vi "field_sweep_2.vi"() -> ()   [LabVIEW 2016]
uses:
  Controls/State.ctl
  Controls/Data.ctl
  <vilib>/Utility/error.llb/DialogType.ctl
  <vilib>/DAQmx/write.llb/DAQmx Write (Analog DBL 1Chan 1Samp).vi
  <vilib>/DAQmx/create/channels.llb/DAQmx Create Channel (AO-Voltage-Basic).vi
  <vilib>/DAQmx/miscellaneous.llb/DAQmx Fill In Error Info.vi
  <instrlib>/niVNA/niVNA.llb/niVNA Fetch Sweep Measurement (DBL).vi
panel:
  in  "Clear button":bool
  in  "Hysteresis":bool caption="Hysteresis On/Off"
  out "DAQ channel Out":tag="DAQ_6363/ao1"
  in  "Averaging Points":i32=10 min=1 max=3201 step=1
  in  "DAQ channel In":tag="DAQ_6363/ao1"
  in  "Exit Button":bool
  in  "IF Bandwidth":dbl(ring)=1000.0 items=["10 Hz"=10.0, "30 Hz"=30.0, "100 Hz"=100.0, "300 Hz"=300.0, "1 KHz"=1000.0, "3 KHz"=3000.0, "10 KHz"=10000.0, "30 KHz"=30000.0]
  in  "Speed (Oe/sec)":dbl=5.0
  in  "Frequency (Hz)":dbl=3000000000.0 min=10000000.0 max=6000000000.0
  in  "Save Button":bool
  out "Status":string="Shutting down...Sweeping field to zero..."
  out "Cursor":cluster{"x":dbl, "y":dbl} {"x" format="%.2f"; "y" format="%.5f"}
  out "VNA Name Out":refnum<k15>="VNA_5630"
  out "Error Out":errorcluster
  in  "Error In (no error)":errorcluster
  in  "Format":i32(ring)=1 items=["Log Magnitude (dB)"=0, "Lin Magnitude"=1, "Phase (deg)"=2, "VSWR"=3, "Group Delay"=6]
  out "SpectrumGraph":cluster{"Old Field":dbl[], "Old Signal":dbl[]}[](graph)
  in  "S-parameter":i32(ring)=1 caption="Measurement" items=["S11", "S21"]
  in  "Start Button":bool
  in  "Stop Button":bool
  in  "Output Power (dBm)":dbl=1.0 min=-25.0 max=5.0 step=0.5
  in  "Number of Points":i32=1000 min=1 max=3201 step=1
  in  "Stop H Field (Oe)":dbl=1500.0 min=-6000.0 max=6000.0 format="%#_6f"
  in  "Start H Field (Oe)":dbl=1000.0 min=-6000.0 max=6000.0 format="%#_6f"
  in  "VNA Name In":refnum<k15>="VNA_5630"
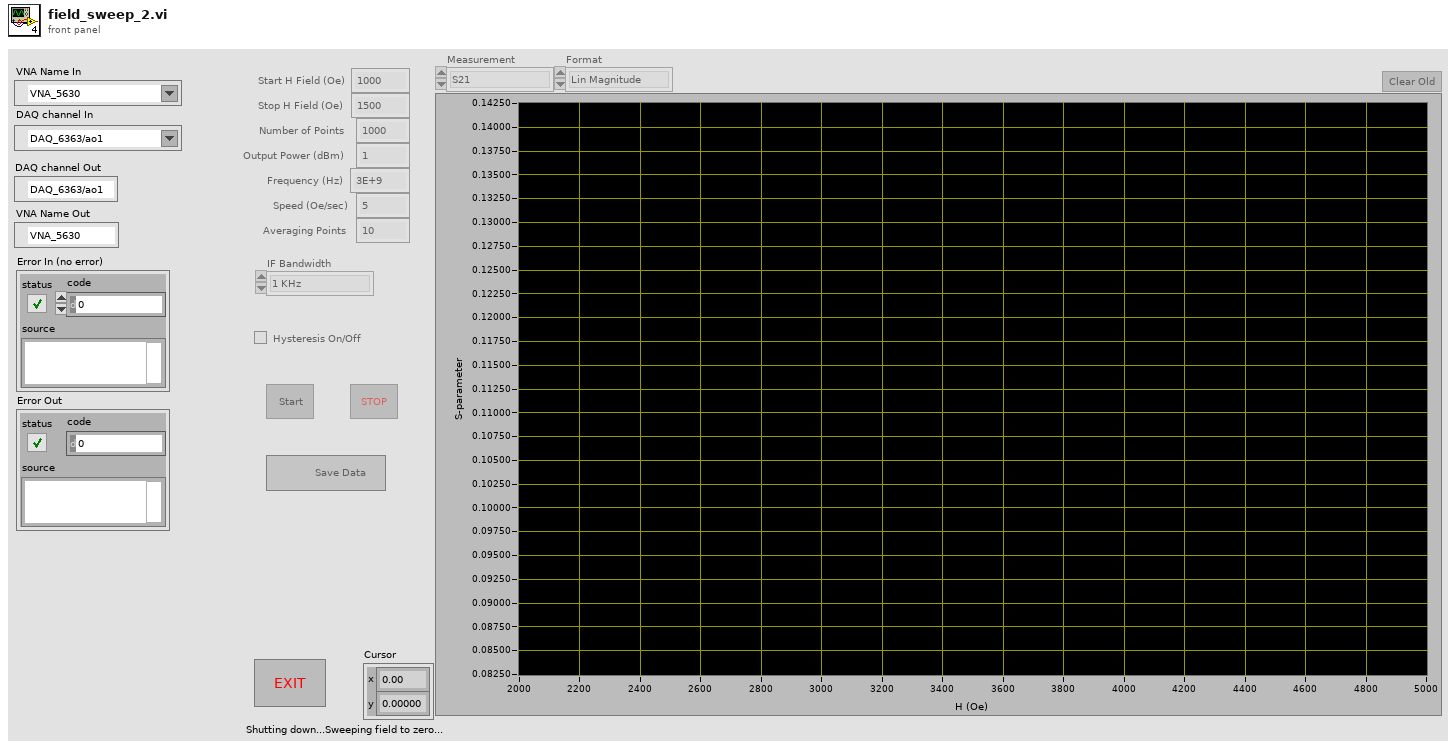
[diagram p1: front panel]
types:
  T1 = typedef "Data.ctl" = cluster{"Field":dbl[], "Signal":dbl[], "Old Field":dbl[], "Old Signal":dbl[]}
  T2 = typedef "State.ctl" = enum16{"Init", "Idle", "Sweeping up", "Sweeping down", "Running", "Running down", "Shutdown"}
  T3 = typedef "DialogType.ctl" = u16
  T4 = typedef "LVPoint32TypeDef.ctl" = cluster{"Horizontal":i32, "Vertical":i32}
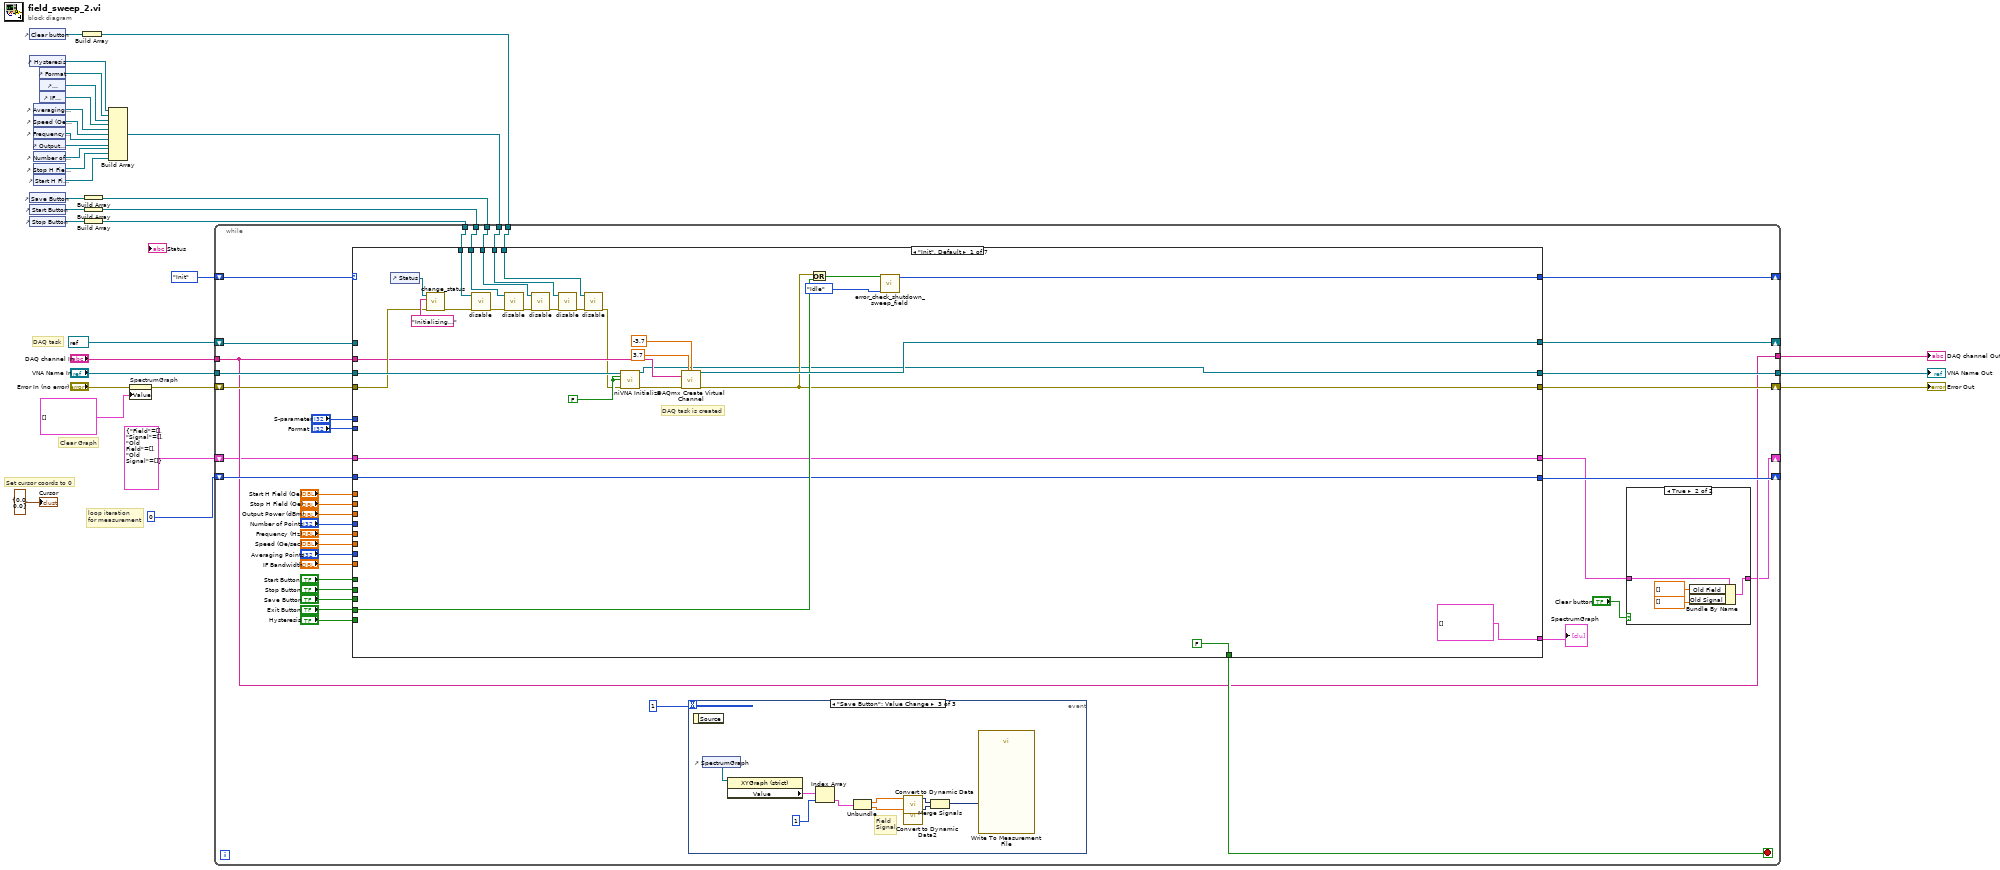
[diagram p0: block diagram]
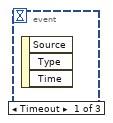
[diagram p3: hidden frame]
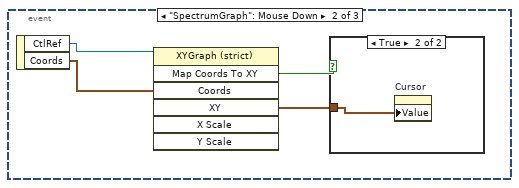
[diagram p4: hidden frame]
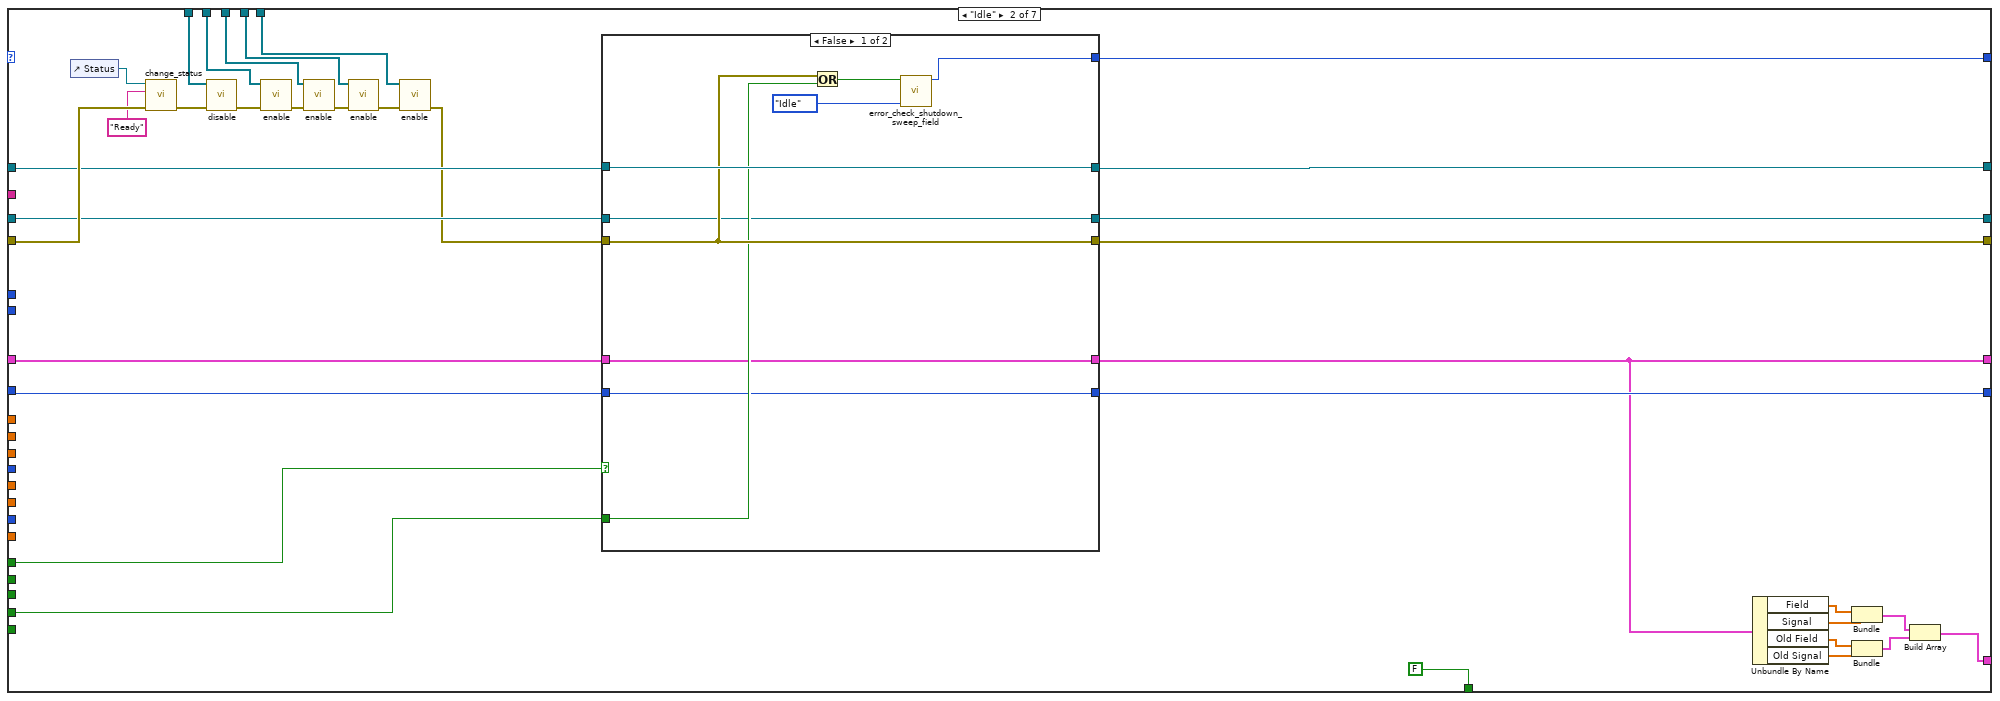
[diagram p6: hidden frame]
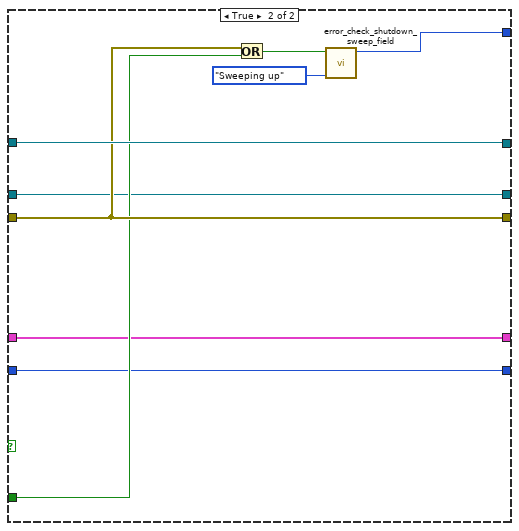
[diagram p7: hidden frame]
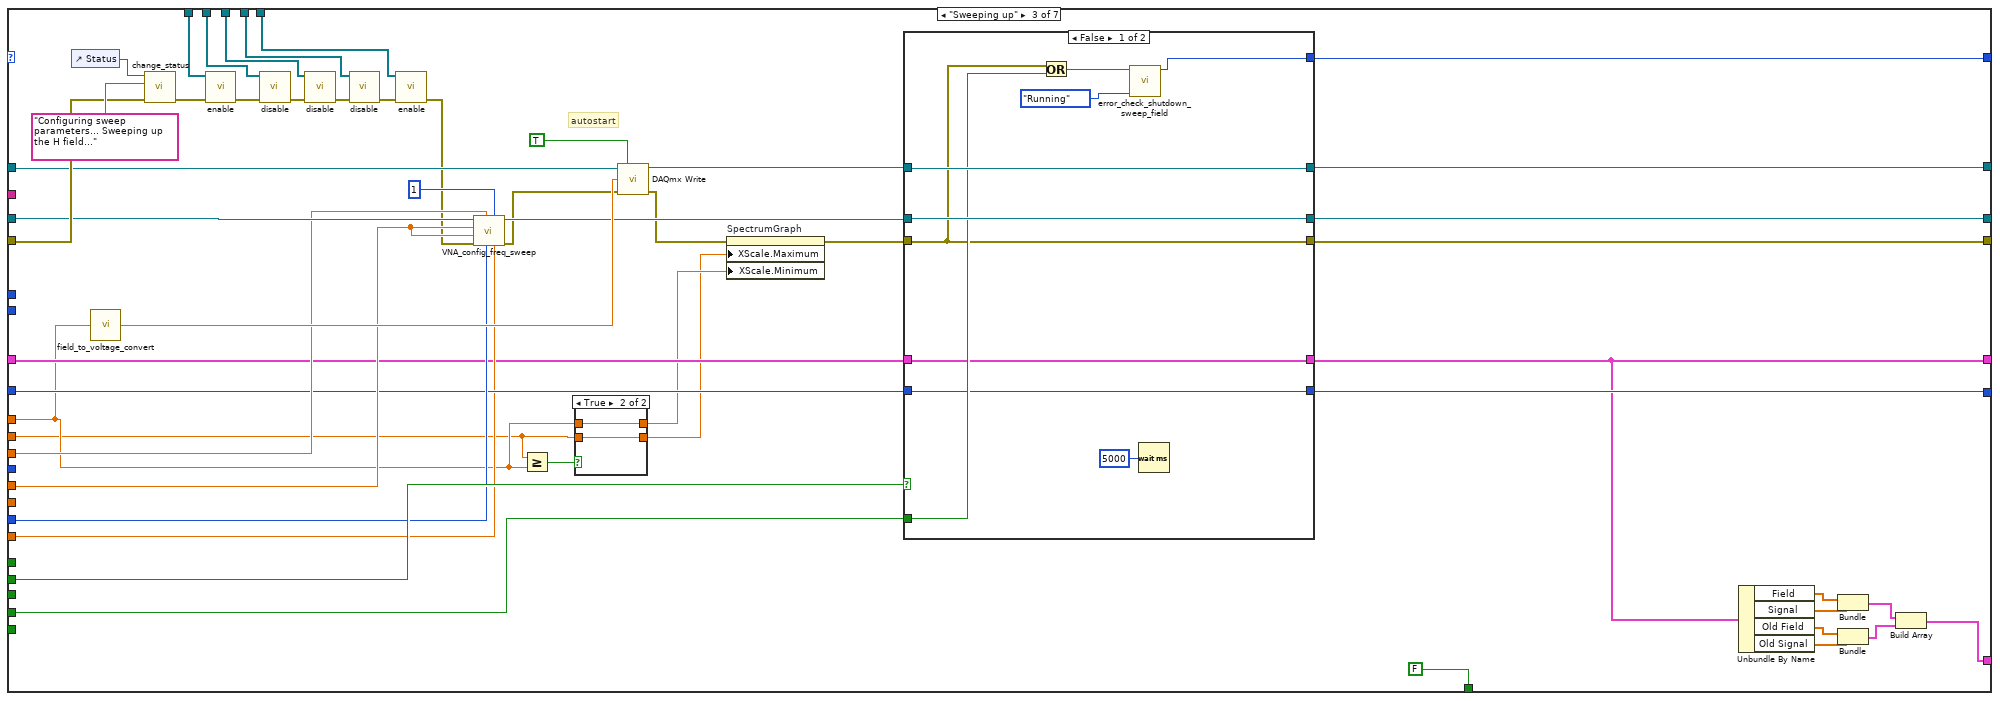
[diagram p8: hidden frame]
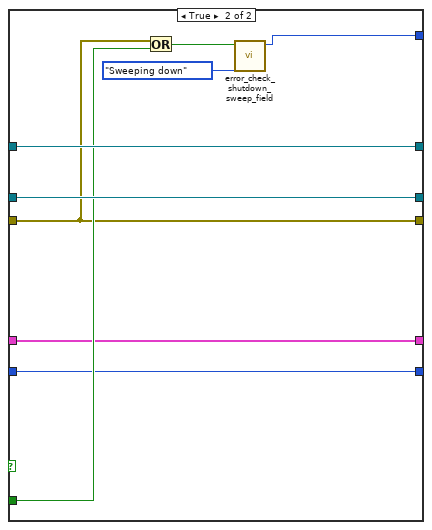
[diagram p10: hidden frame]
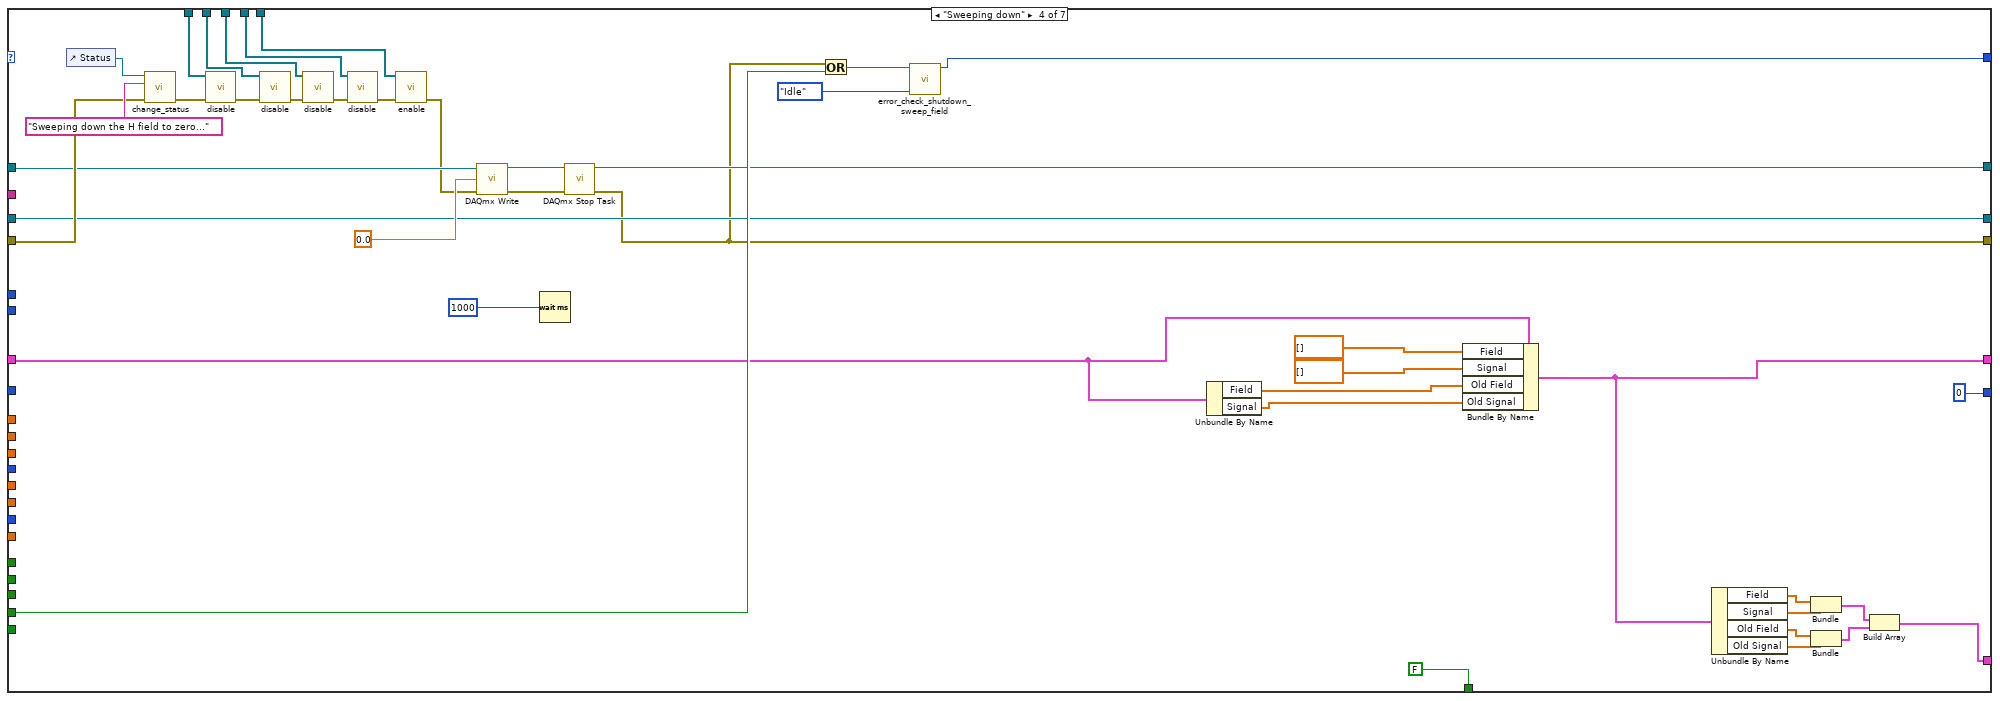
[diagram p11: hidden frame]
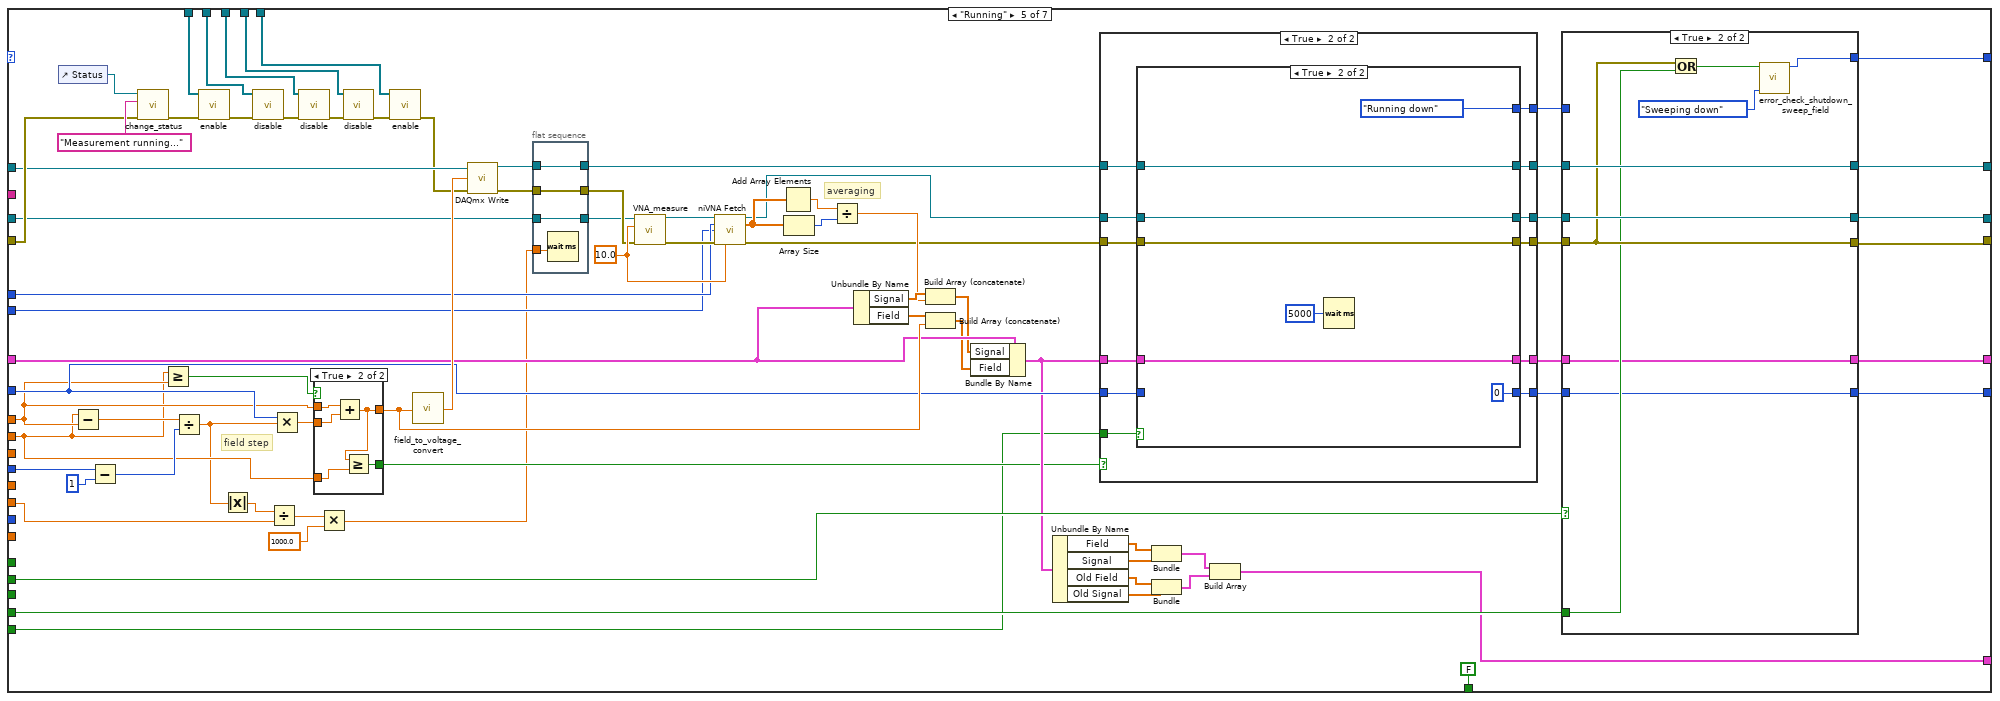
[diagram p12: hidden frame]
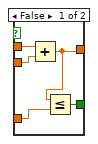
[diagram p13: hidden frame]
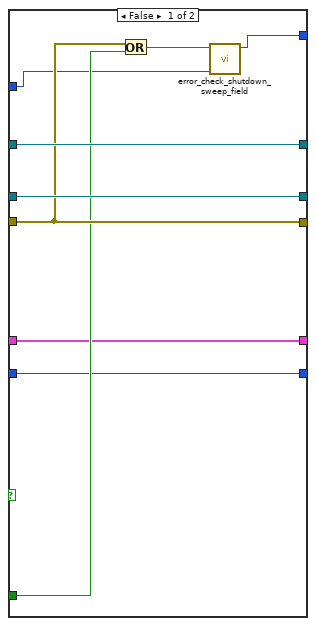
[diagram p14: hidden frame]
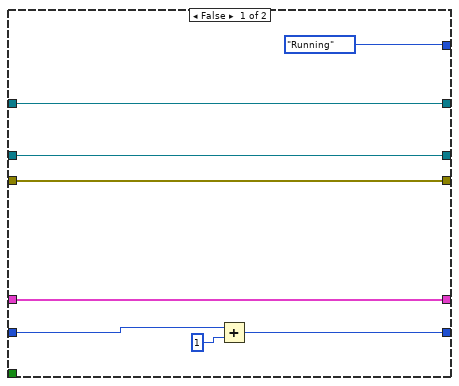
[diagram p15: hidden frame]
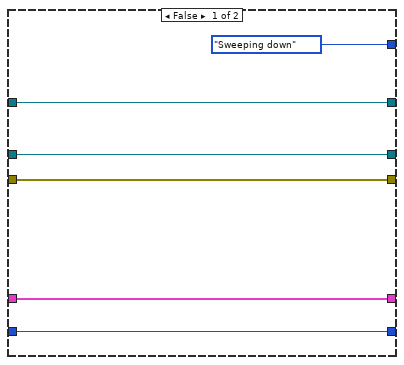
[diagram p16: hidden frame]
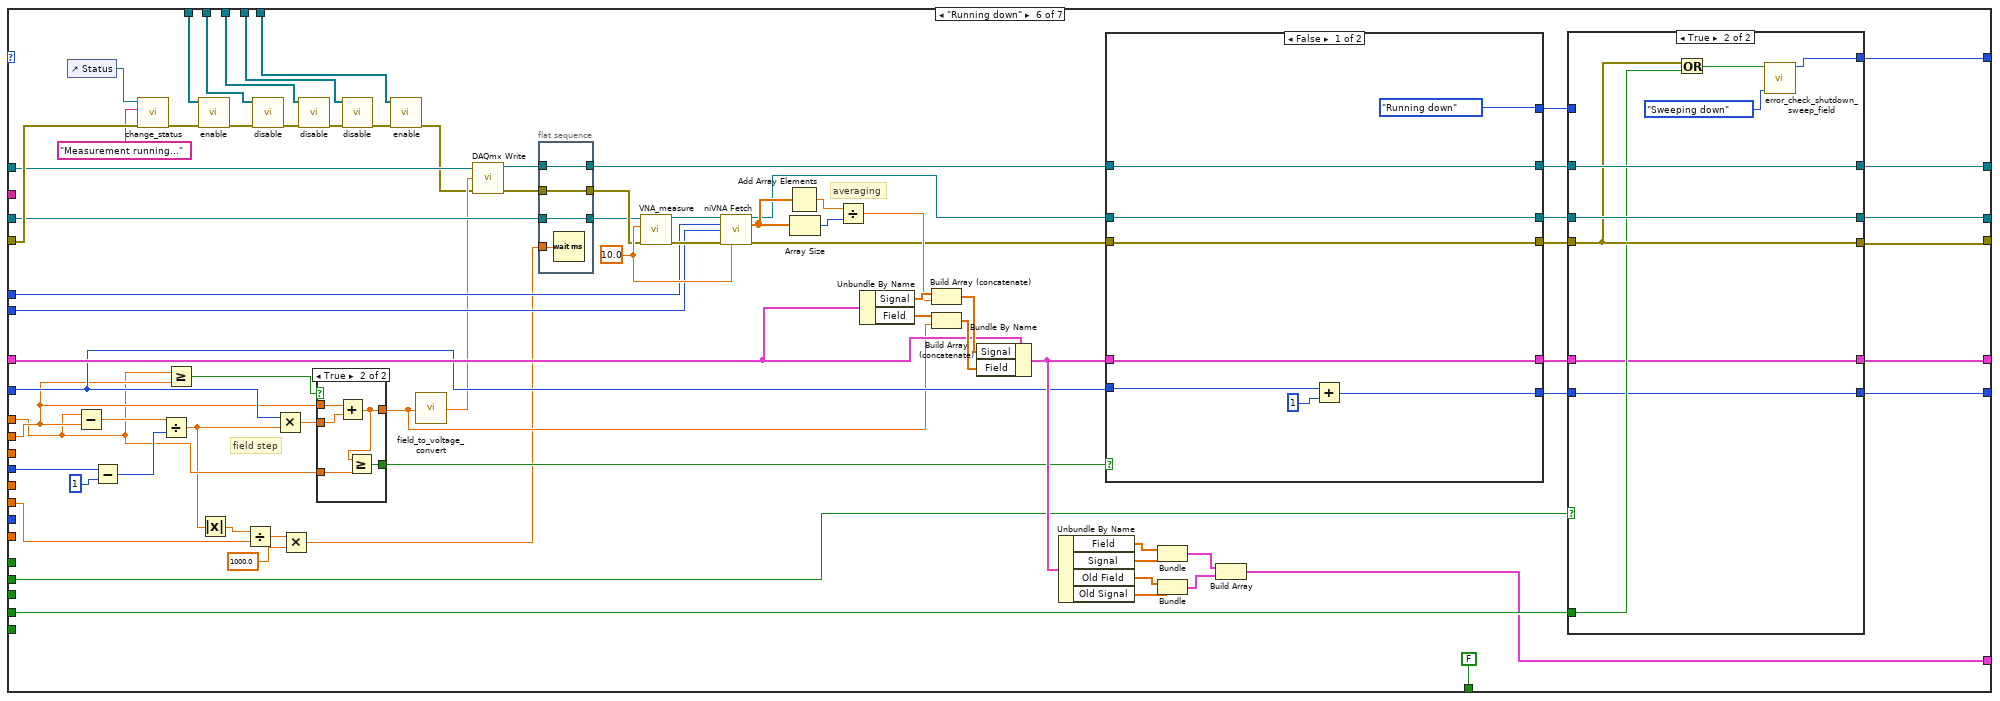
[diagram p17: hidden frame]
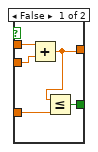
[diagram p18: hidden frame]
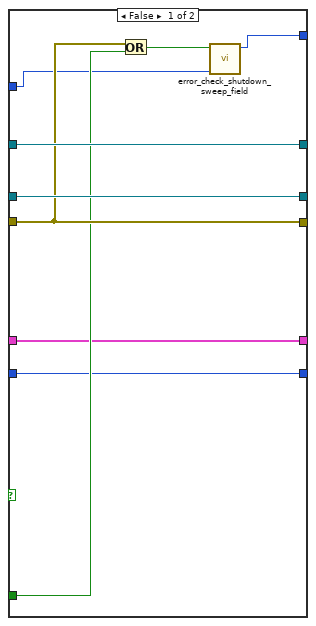
[diagram p19: hidden frame]
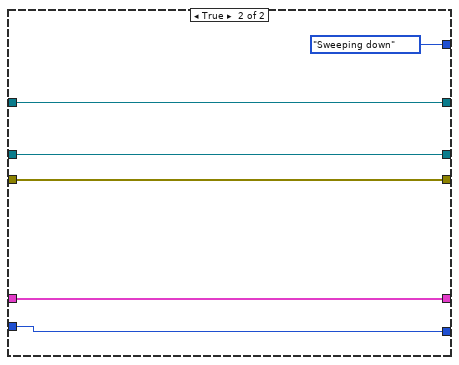
[diagram p20: hidden frame]
diagram:
  # "loop iteration\nfor measurement"
  # "DAQ task"
  # "Set cursor coords to 0"
  # "Clear Graph"
  n1 = control-ref of="Clear button"() -> (w2:refnum<vi>)
  n2 = control-ref of="Hysteresis"() -> (w3:refnum<vi>)
  n3 = control-ref of="Save Button"() -> (w16:refnum<vi>)
  n4 = control-ref of="Start Button"() -> (w24:refnum<vi>)
  n5 = control-ref of="Stop Button"() -> (w23:refnum<vi>)
  n6 = control-ref of="Averaging Points"() -> (w13:refnum<vi>)
  n7 = control-ref of="Speed (Oe/sec)"() -> (w30:refnum<vi>)
  n8 = control-ref of="Frequency (Hz)"() -> (w29:refnum<vi>)
  n9 = control-ref of="Output Power (dBm)"() -> (w28:refnum<vi>)
  n10 = control-ref of="Number of Points"() -> (w27:refnum<vi>)
  n11 = control-ref of="Stop H Field (Oe)"() -> (w26:refnum<vi>)
  n12 = control-ref of="Start H Field (Oe)"() -> (w25:refnum<vi>)
  n13 = control-ref of="Format"() -> (w4:refnum<vi>)
  n14 = control-ref of="S-parameter"() -> (w5:refnum<vi>)
  n15 = control-ref of="IF Bandwidth"() -> (w31:refnum<vi>)
  n16 = Build Array(w2) -> (w1:refnum<vi>[])
  n17 = Build Array(w16) -> (w15:refnum<vi>[])
  n18 = Build Array(w24) -> (w21:refnum<vi>[])
  n19 = Build Array(w23) -> (w20:refnum<vi>[])
  n20 = Build Array(w3, w4, w5, w31, w13, w30, w29, w28, w27, w26, w25) -> (w22:refnum<vi>[])
  n21 = property on="SpectrumGraph" class="XYGraph (strict)"(error in="Error In (no error)", "Value"=cluster{"Old Field":dbl[], "Old Signal":dbl[]}[] [] ("SpectrumGraph")) -> (error out=w9:errorcluster)  [unwired: 1 in, 1 out]
  n22 = while {
    shift-right: [w66] -> _
    shift-left: State."Init" -> [w71]
    shift-right: [w46] -> _
    shift-left: 0 -> [w48]
    tunnel: w22 -> [w70]
    tunnel: w21 -> [w69]
    tunnel: w20 -> [w68]
    tunnel: "VNA Name In" -> [w67]
    tunnel: "DAQ channel In" -> [w45]
    shift-right: [w65] -> w6
    shift-left: w9 -> [w64]
    shift-right: [w63] -> _
    shift-left: refnum<k21> refnum ("task in") -> [w62]
    tunnel: w15 -> [w61]
    tunnel: [w49] -> w12
    shift-right: [w35] -> _
    shift-left: T1 {"Field"=[], "Signal"=[], "Old Field"=[], "Old Signal"=[]} ("Cluster") -> [w42]
    tunnel: [w45] -> w11
    tunnel: w1 -> [w34]
    stop <- w56 stop-if-true
    n23 = case shown="\"Init\", Default" w71 {
      tunnel: w70 -> [w106 w152 w216 w280 w359 w500 w585]
      tunnel: w69 -> [w119 w154 w218 w278 w361 w502 w587]
      tunnel: w68 -> [w121 w155 w219 w277 w363 w503 w588]
      tunnel: w67 -> [w114 w142 w205 w273 w334 w472 w570]
      tunnel: w64 -> [w113 w147 w214 w283 w357 w506 w583]
      tunnel: [w102 w139 w207 w274 w318 w456 State."Shutdown"] -> w66
      tunnel: w45 -> [w109 _ _ _ _ _ _]
      tunnel: [w101 w143 w212 w266 w324 w458 w578] -> w65
      tunnel: [w108 w140 w210 w268 w328 w457 w579] -> w63
      tunnel: w62 -> [_ w141 w192 w281 w356 w473 w573]
      tunnel: w61 -> [w107 w153 w217 w279 w360 w501 w586]
      tunnel: "Start Button" -> [_ w144 _ _ _ _ _]
      tunnel: "Stop Button" -> [_ _ w213 _ w323 w469 _]
      tunnel: "Save Button" -> [_ _ _ _ _ _ _]
      tunnel: "Exit Button" -> [w103 w138 w206 w275 w322 w462 _]
      tunnel: [FALSE FALSE FALSE FALSE FALSE FALSE TRUE] -> w56
      tunnel: "Start H Field (Oe)" -> [_ _ w188 _ w304 w445 _]
      tunnel: "Stop H Field (Oe)" -> [_ _ w187 _ w302 w446 _]
      tunnel: "Output Power (dBm)" -> [_ _ w202 _ _ _ _]
      tunnel: "Number of Points" -> [_ _ _ _ w345 w449 _]
      tunnel: "Frequency (Hz)" -> [_ _ w203 _ _ _ _]
      tunnel: "Speed (Oe/sec)" -> [_ _ _ _ w346 w438 _]
      tunnel: [w99 w137 w211 w273 w326 w459 w580] -> w49
      tunnel: w48 -> [w98 w135 w200 _ w330 w450 w568]
      tunnel: "Averaging Points" -> [_ _ w201 _ _ _ _]
      tunnel: [w98 w136 w199 0 w320 w460 w568] -> w46
      tunnel: "IF Bandwidth" -> [_ _ w195 _ _ _ _]
      tunnel: [w96 w125 w177 w251 w312 w461 T1 {"Field"=[], "Signal"=[], "Old Field"=[], "Old Signal"=[]} ("Cluster")] -> w36
      tunnel: w42 -> [w96 w133 w193 w262 w316 w468 _]
      tunnel: "Hysteresis" -> [_ _ _ _ w300 _ _]
      tunnel: "S-parameter" -> [_ _ _ _ w299 w471 _]
      tunnel: "Format" -> [_ _ _ _ w298 w470 _]
      tunnel: [cluster{"Old Field":dbl[], "Old Signal":dbl[]}[] [] w126 w178 w252 w297 w444 cluster{"Old Field":dbl[], "Old Signal":dbl[]}[] []] -> w38
      tunnel: w34 -> [w92 w123 w175 w249 w289 w434 w558]
      frame "Init", Default {
        w115 = FALSE ("id query")
        # "DAQ task is created"
        n24 = control-ref of="Status"() -> (w117:refnum<vi>)
        n25 = call "change_status.vi"("error in (no error)"=w113, "String"="Initializing...", "String in"=w117) -> ("error out"=w118:errorcluster)  [unwired: 8 in]
        n26 = call "disable.vi"("error in (no error)"=w118, "Array"=w121) -> ("error out"=w120:errorcluster)  [unwired: 9 in]
        n27 = call "disable.vi"("error in (no error)"=w120, "Array"=w119) -> ("error out"=w105:errorcluster)  [unwired: 9 in]
        n28 = call "disable.vi"("error in (no error)"=w105, "Array"=w107) -> ("error out"=w104:errorcluster)  [unwired: 9 in]
        n29 = call "disable.vi"("error in (no error)"=w104, "Array"=w106) -> ("error out"=w93:errorcluster)  [unwired: 9 in]
        n30 = call "disable.vi"("error in (no error)"=w93, "Array"=w92) -> ("error out"=w91:errorcluster)  [unwired: 9 in]
        n31 = call <instrlib>:"niVNA Initialize.vi"("resource name"=w114, "id query"=w115, "reset"=w115, "error in"=w91) -> ("instrument handle"=w99:refnum<k15>, "error out"=w112:errorcluster)  [unwired: 10 in]
        n32 = call-poly <vilib>:"DAQmx Create Virtual Channel.vi"("maximum value"=3.7, "minimum value"=-3.7, "physical channels"=w109, "error in"=w112) -> ("task out"=w108:refnum<k21>, "error out"=w101:errorcluster)  [unwired: 10 in]
        n33 = Or(x=w101, y=w103) -> (x .or. y?=w100:bool)
        n34 = call "error_check_shutdown_sweep_field.vi"("State In"=State."Idle", "Boolean"=w100) -> ("State Out"=w102:T2)  [unwired: 9 in]
      }
      frame "Idle" {
        n35 = control-ref of="Status"() -> (w146:refnum<vi>)
        n36 = call "change_status.vi"("error in (no error)"=w147, "String"="Ready", "String in"=w146) -> ("error out"=w148:errorcluster)  [unwired: 8 in]
        n37 = call "disable.vi"("error in (no error)"=w148, "Array"=w155) -> ("error out"=w151:errorcluster)  [unwired: 9 in]
        n38 = call "enable.vi"("error in (no error)"=w151, "Array"=w154) -> ("error out"=w150:errorcluster)  [unwired: 9 in]
        n39 = call "enable.vi"("error in (no error)"=w150, "Array"=w153) -> ("error out"=w149:errorcluster)  [unwired: 9 in]
        n40 = call "enable.vi"("error in (no error)"=w149, "Array"=w152) -> ("error out"=w124:errorcluster)  [unwired: 9 in]
        n41 = call "enable.vi"("error in (no error)"=w124, "Array"=w123) -> ("error out"=w122:errorcluster)  [unwired: 9 in]
        n42 = case shown="False" w144 {
          tunnel: w122 -> [w161 w171]
          tunnel: [w161 w171] -> w143
          tunnel: w142 -> [w159 w168]
          tunnel: w141 -> [w164 w173]
          tunnel: [w164 w173] -> w140
          tunnel: [w162 w169] -> w139
          tunnel: w138 -> [w160 w170]
          tunnel: [w159 w168] -> w137
          tunnel: [w158 w167] -> w136
          tunnel: w135 -> [w158 w167]
          tunnel: w133 -> [w157 w166]
          tunnel: [w157 w166] -> w125
          frame False {
            n43 = Or(x=w161, y=w160) -> (x .or. y?=w163:bool)
            n44 = call "error_check_shutdown_sweep_field.vi"("State In"=State."Idle", "Boolean"=w163) -> ("State Out"=w162:T2)  [unwired: 9 in]
          }
          frame True {
            n45 = Or(x=w171, y=w170) -> (x .or. y?=w172:bool)
            n46 = call "error_check_shutdown_sweep_field.vi"("State In"=State."Sweeping up", "Boolean"=w172) -> ("State Out"=w169:T2)  [unwired: 9 in]
          }
        }
        n47 = Unbundle By Name(w125) -> ("Field"=w132:dbl[], "Signal"=w131:dbl[], "Old Field"=w130:dbl[], "Old Signal"=w129:dbl[])
        n48 = Bundle("Field"=w132, "Signal"=w131) -> (w128:cluster{"Field":dbl[], "Signal":dbl[]})  [unwired: 1 in]
        n49 = Bundle("Old Field"=w130, "Old Signal"=w129) -> (w127:cluster{"Old Field":dbl[], "Old Signal":dbl[]})  [unwired: 1 in]
        n50 = Build Array(w128, w127) -> (w126:cluster{"Old Field":dbl[], "Old Signal":dbl[]}[])
      }
      frame "Sweeping up" {
        # "autostart"
        n51 = control-ref of="Status"() -> (w215:refnum<vi>)
        n52 = call "field_to_voltage_convert.vi"("Start H Field (Oe)"=w188) -> ("Numeric"=w208:dbl)
        n53 = call "change_status.vi"("error in (no error)"=w214, "String"="Configuring sweep parameters... Sweeping up the H field...", "String in"=w215) -> ("error out"=w223:errorcluster)  [unwired: 8 in]
        n54 = call "enable.vi"("error in (no error)"=w223, "Array"=w219) -> ("error out"=w222:errorcluster)  [unwired: 9 in]
        n55 = call "disable.vi"("error in (no error)"=w222, "Array"=w218) -> ("error out"=w221:errorcluster)  [unwired: 9 in]
        n56 = call "disable.vi"("error in (no error)"=w221, "Array"=w217) -> ("error out"=w220:errorcluster)  [unwired: 9 in]
        n57 = call "disable.vi"("error in (no error)"=w220, "Array"=w216) -> ("error out"=w176:errorcluster)  [unwired: 9 in]
        n58 = call "enable.vi"("error in (no error)"=w176, "Array"=w175) -> ("error out"=w174:errorcluster)  [unwired: 9 in]
        n59 = call "VNA_config_freq_sweep.vi"("IF Bandwidth"=w195, "Averaging"=1, "Number of Points"=w201, "Output Power"=w202, "error in (no error)"=w174, "Stop Frequency"=w203, "Start Frequency"=w203, "Resource Name In"=w205) -> ("error out"=w191:errorcluster, "Resource Name Out"=w204:refnum<k15>)  [unwired: 2 in]
        n60 = Greater Or Equal?(x=w187, y=w188) -> (x >= y?=w189:bool)
        n61 = case shown="True" w189 {
          tunnel: w188 -> [w226 w228]
          tunnel: w187 -> [w225 w227]
          tunnel: [w225 w228] -> w186
          tunnel: [w226 w227] -> w185
          frame False {
          }
          frame True {
          }
        }
        n62 = call-poly <vilib>:"DAQmx Write.vi"("task/channels in"=w192, "auto start"=TRUE, "data"=w208, "error in"=w191) -> ("task out"=w209:refnum<k21>, "error out"=w197:errorcluster)  [unwired: 9 in, 1 out]
        n63 = property on="SpectrumGraph" class="XYGraph (strict)"(error in=w197, "XScale.Maximum"=w185, "XScale.Minimum"=w186) -> (error out=w196:errorcluster)  [unwired: 1 in, 1 out]
        n64 = case shown="False" w213 {
          tunnel: w196 -> [w233 w242]
          tunnel: w209 -> [w238 w246]
          tunnel: w204 -> [w237 w247]
          tunnel: [w233 w242] -> w212
          tunnel: [w237 w247] -> w211
          tunnel: [w238 w246] -> w210
          tunnel: [w235 w244] -> w207
          tunnel: w206 -> [w234 w243]
          tunnel: w200 -> [w231 w241]
          tunnel: [w231 w241] -> w199
          tunnel: w193 -> [w230 w240]
          tunnel: [w230 w240] -> w177
          frame False {
            n65 = Or(x=w233, y=w234) -> (x .or. y?=w236:bool)
            n66 = call "error_check_shutdown_sweep_field.vi"("State In"=State."Running", "Boolean"=w236) -> ("State Out"=w235:T2)  [unwired: 9 in]
            n67 = Wait (ms)(milliseconds to wait=u32 5000) -> ()  [unwired: 1 out]
          }
          frame True {
            n68 = Or(x=w242, y=w243) -> (x .or. y?=w245:bool)
            n69 = call "error_check_shutdown_sweep_field.vi"("State In"=State."Sweeping down", "Boolean"=w245) -> ("State Out"=w244:T2)  [unwired: 9 in]
          }
        }
        n70 = Unbundle By Name(w177) -> ("Field"=w184:dbl[], "Signal"=w183:dbl[], "Old Field"=w182:dbl[], "Old Signal"=w181:dbl[])
        n71 = Bundle("Field"=w184, "Signal"=w183) -> (w180:cluster{"Field":dbl[], "Signal":dbl[]})  [unwired: 1 in]
        n72 = Bundle("Old Field"=w182, "Old Signal"=w181) -> (w179:cluster{"Old Field":dbl[], "Old Signal":dbl[]})  [unwired: 1 in]
        n73 = Build Array(w180, w179) -> (w178:cluster{"Old Field":dbl[], "Old Signal":dbl[]}[])
      }
      frame "Sweeping down" {
        n74 = control-ref of="Status"() -> (w272:refnum<vi>)
        n75 = call "change_status.vi"("error in (no error)"=w283, "String"="Sweeping down the H field to zero...", "String in"=w272) -> ("error out"=w287:errorcluster)  [unwired: 8 in]
        n76 = call "disable.vi"("error in (no error)"=w287, "Array"=w277) -> ("error out"=w286:errorcluster)  [unwired: 9 in]
        n77 = call "disable.vi"("error in (no error)"=w286, "Array"=w278) -> ("error out"=w285:errorcluster)  [unwired: 9 in]
        n78 = call "disable.vi"("error in (no error)"=w285, "Array"=w279) -> ("error out"=w284:errorcluster)  [unwired: 9 in]
        n79 = call "disable.vi"("error in (no error)"=w284, "Array"=w280) -> ("error out"=w250:errorcluster)  [unwired: 9 in]
        n80 = call "enable.vi"("error in (no error)"=w250, "Array"=w249) -> ("error out"=w248:errorcluster)  [unwired: 9 in]
        n81 = call-poly <vilib>:"DAQmx Write.vi"("task/channels in"=w281, "data"=0.0, "error in"=w248) -> ("task out"=w269:refnum<k21>, "error out"=w267:errorcluster)  [unwired: 10 in, 1 out]
        n82 = Wait (ms)(milliseconds to wait=u32 1000) -> ()  [unwired: 1 out]
        n83 = call <vilib>:"DAQmx Stop Task.vi"("task/channels in"=w269, "error in"=w267) -> ("task out"=w268:refnum<k21>, "error out"=w266:errorcluster)  [unwired: 12 in]
        n84 = Or(x=w266, y=w275) -> (x .or. y?=w276:bool)
        n85 = call "error_check_shutdown_sweep_field.vi"("State In"=State."Idle", "Boolean"=w276) -> ("State Out"=w274:T2)  [unwired: 9 in]
        n86 = Unbundle By Name(w262) -> ("Field"=w261:dbl[], "Signal"=w260:dbl[])
        n87 = Bundle By Name(cluster=w262, "Field"=dbl[] [], "Signal"=dbl[] [], "Old Field"=w261, "Old Signal"=w260) -> (w251:T1)
        n88 = Unbundle By Name(w251) -> ("Field"=w258:dbl[], "Signal"=w257:dbl[], "Old Field"=w256:dbl[], "Old Signal"=w255:dbl[])
        n89 = Bundle("Field"=w258, "Signal"=w257) -> (w254:cluster{"Field":dbl[], "Signal":dbl[]})  [unwired: 1 in]
        n90 = Bundle("Old Field"=w256, "Old Signal"=w255) -> (w253:cluster{"Old Field":dbl[], "Old Signal":dbl[]})  [unwired: 1 in]
        n91 = Build Array(w254, w253) -> (w252:cluster{"Old Field":dbl[], "Old Signal":dbl[]}[])
      }
      frame "Running" {
        w352 = 10.0 ("timeout")
        # "averaging"
        # "field step"
        n92 = control-ref of="Status"() -> (w358:refnum<vi>)
        n93 = Subtract(x=w302, y=w304) -> (x-y=w340:dbl)
        n94 = Subtract(x=w345, y=1) -> (x-y=w354:i32)
        n95 = call "change_status.vi"("error in (no error)"=w357, "String"="Measurement running...", "String in"=w358) -> ("error out"=w364:errorcluster)  [unwired: 8 in]
        n96 = Greater Or Equal?(x=w302, y=w304) -> (x >= y?=w303:bool)
        n97 = Divide(x=w340, y=w354) -> (x/y=w293:dbl)
        n98 = call "enable.vi"("error in (no error)"=w364, "Array"=w363) -> ("error out"=w367:errorcluster)  [unwired: 9 in]
        n99 = Absolute Value(x=w293) -> (abs(x)=w292:dbl)
        n100 = call "disable.vi"("error in (no error)"=w367, "Array"=w361) -> ("error out"=w366:errorcluster)  [unwired: 9 in]
        n101 = Divide(x=w292, y=w346) -> (x/y=w296:dbl)
        n102 = Multiply(x=w330, y=w293) -> (x*y=w353:dbl)
        n103 = call "disable.vi"("error in (no error)"=w366, "Array"=w360) -> ("error out"=w365:errorcluster)  [unwired: 9 in]
        n104 = case shown="True" w303 {
          tunnel: w353 -> [w371 w377]
          tunnel: w304 -> [w372 w376]
          tunnel: [w369 w374] -> w336
          tunnel: w302 -> [w370 w373]
          tunnel: [w368 w375] -> w301
          frame False {
            n105 = Add(x=w372, y=w371) -> (x+y=w369:dbl)
            n106 = Less Or Equal?(x=w369, y=w370) -> (x <= y?=w368:bool)
          }
          frame True {
            n107 = Add(x=w376, y=w377) -> (x+y=w374:dbl)
            n108 = Greater Or Equal?(x=w374, y=w373) -> (x >= y?=w375:bool)
          }
        }
        n109 = Multiply(x=w296, y=1000.0) -> (x*y=w294:dbl)
        n110 = call "disable.vi"("error in (no error)"=w365, "Array"=w359) -> ("error out"=w291:errorcluster)  [unwired: 9 in]
        n111 = call "enable.vi"("error in (no error)"=w291, "Array"=w289) -> ("error out"=w290:errorcluster)  [unwired: 9 in]
        n112 = call "field_to_voltage_convert.vi"("Start H Field (Oe)"=w336) -> ("Numeric"=w341:dbl)
        n113 = call-poly <vilib>:"DAQmx Write.vi"("task/channels in"=w356, "data"=w341, "error in"=w290) -> ("task out"=w344:refnum<k21>, "error out"=w343:errorcluster)  [unwired: 10 in, 1 out]
        n114 = flat-sequence {
          tunnel: w344 -> [w432]
          tunnel: [w432] -> w335
          tunnel: w343 -> [w431]
          tunnel: [w431] -> w342
          tunnel: w334 -> [w430]
          tunnel: [w430] -> w333
          tunnel: w294 -> [w429]
          frame #0 {
            n115 = Wait (ms)(milliseconds to wait=w429) -> ()  [unwired: 1 out]
          }
        }
        n116 = call "VNA_measure.vi"("error in (no error)"=w342, "timeout"=w352, "Resource Name In"=w333) -> ("error out"=w351:errorcluster, "Resource Name Out"=w350:refnum<k15>)  [unwired: 7 in]
        n117 = call-poly <instrlib>:"niVNA Fetch.vi"("instrument handle"=w350, "measurement"=w299, "format"=w298, "error in"=w351, "timeout"=w352) -> ("instrument handle out"=w332:refnum<k15>, "data"=w349:dbl[], "error out"=w331:errorcluster)  [unwired: 7 in, 1 out]
        n118 = Add Array Elements(numeric array=w349) -> (sum=w348:dbl)
        n119 = Array Size(array=w349) -> (size(s)=w347:i32)
        n120 = Divide(x=w348, y=w347) -> (x/y=w338:dbl)
        n121 = Unbundle By Name(w316) -> ("Signal"=w339:dbl[], "Field"=w337:dbl[])
        n122 = Build Array (concatenate)(w339, w338) -> (w315:dbl[])
        n123 = Build Array (concatenate)(w337, w336) -> (w314:dbl[])
        n124 = Bundle By Name(cluster=w316, "Signal"=w315, "Field"=w314) -> (w311:T1)
        n125 = Unbundle By Name(w311) -> ("Field"=w310:dbl[], "Signal"=w309:dbl[], "Old Field"=w308:dbl[], "Old Signal"=w307:dbl[])
        n126 = case shown="True" w301 {
          tunnel: [State."Running" w415] -> w319
          tunnel: w335 -> [w402 w405]
          tunnel: [w402 w404] -> w329
          tunnel: w332 -> [w401 w407]
          tunnel: [w401 w406] -> w327
          tunnel: w331 -> [w400 w409]
          tunnel: [w400 w408] -> w325
          tunnel: w330 -> [w399 w414]
          tunnel: [w397 w412] -> w321
          tunnel: w311 -> [w396 w411]
          tunnel: [w396 w410] -> w313
          tunnel: w300 -> [_ w413]
          frame False {
            n127 = Add(x=w399, y=1) -> (x+y=w397:i32)
          }
          frame True {
            n128 = case shown="True" w413 {
              tunnel: [State."Sweeping down" State."Running down"] -> w415
              tunnel: w414 -> [w420 _]
              tunnel: [w420 0] -> w412
              tunnel: w411 -> [w419 w425]
              tunnel: [w419 w425] -> w410
              tunnel: w409 -> [w418 w423]
              tunnel: [w418 w423] -> w408
              tunnel: w407 -> [w417 w426]
              tunnel: [w417 w426] -> w406
              tunnel: w405 -> [w416 w427]
              tunnel: [w416 w427] -> w404
              frame False {
              }
              frame True {
                n129 = Wait (ms)(milliseconds to wait=u32 5000) -> ()  [unwired: 1 out]
              }
            }
          }
        }
        n130 = Bundle("Field"=w310, "Signal"=w309) -> (w306:cluster{"Field":dbl[], "Signal":dbl[]})  [unwired: 1 in]
        n131 = Bundle("Old Field"=w308, "Old Signal"=w307) -> (w305:cluster{"Old Field":dbl[], "Old Signal":dbl[]})  [unwired: 1 in]
        n132 = Build Array(w306, w305) -> (w297:cluster{"Old Field":dbl[], "Old Signal":dbl[]}[])
        n133 = case shown="True" w323 {
          tunnel: [w385 w394] -> w318
          tunnel: w329 -> [w384 w393]
          tunnel: [w384 w393] -> w328
          tunnel: w327 -> [w383 w392]
          tunnel: [w383 w392] -> w326
          tunnel: w325 -> [w382 w391]
          tunnel: [w382 w391] -> w324
          tunnel: w322 -> [w381 w390]
          tunnel: w321 -> [w380 w389]
          tunnel: [w380 w389] -> w320
          tunnel: w319 -> [w378 _]
          tunnel: [w379 w388] -> w312
          tunnel: w313 -> [w379 w388]
          frame False {
            n134 = Or(x=w382, y=w381) -> (x .or. y?=w386:bool)
            n135 = call "error_check_shutdown_sweep_field.vi"("State In"=w378, "Boolean"=w386) -> ("State Out"=w385:T2)  [unwired: 9 in]
          }
          frame True {
            n136 = Or(x=w391, y=w390) -> (x .or. y?=w395:bool)
            n137 = call "error_check_shutdown_sweep_field.vi"("State In"=State."Sweeping down", "Boolean"=w395) -> ("State Out"=w394:T2)  [unwired: 9 in]
          }
        }
      }
      frame "Running down" {
        w499 = 10.0 ("timeout")
        # "field step"
        # "averaging"
        n138 = control-ref of="Status"() -> (w505:refnum<vi>)
        n139 = Subtract(x=w445, y=w446) -> (x-y=w452:dbl)
        n140 = Subtract(x=w449, y=1) -> (x-y=w454:i32)
        n141 = call "change_status.vi"("error in (no error)"=w506, "String"="Measurement running...", "String in"=w505) -> ("error out"=w507:errorcluster)  [unwired: 8 in]
        n142 = Divide(x=w452, y=w454) -> (x/y=w437:dbl)
        n143 = Greater Or Equal?(x=w445, y=w446) -> (x >= y?=w451:bool)
        n144 = call "enable.vi"("error in (no error)"=w507, "Array"=w503) -> ("error out"=w510:errorcluster)  [unwired: 9 in]
        n145 = Absolute Value(x=w437) -> (abs(x)=w436:dbl)
        n146 = Divide(x=w436, y=w438) -> (x/y=w441:dbl)
        n147 = call "disable.vi"("error in (no error)"=w510, "Array"=w502) -> ("error out"=w509:errorcluster)  [unwired: 9 in]
        n148 = Multiply(x=w450, y=w437) -> (x*y=w453:dbl)
        n149 = Multiply(x=w441, y=1000.0) -> (x*y=w439:dbl)
        n150 = call "disable.vi"("error in (no error)"=w509, "Array"=w501) -> ("error out"=w508:errorcluster)  [unwired: 9 in]
        n151 = case shown="True" w451 {
          tunnel: w453 -> [w515 w520]
          tunnel: [w514 w518] -> w447
          tunnel: [w513 w519] -> w448
          tunnel: w446 -> [w512 w516]
          tunnel: w445 -> [w511 w517]
          frame False {
            n152 = Add(x=w512, y=w515) -> (x+y=w514:dbl)
            n153 = Less Or Equal?(x=w514, y=w511) -> (x <= y?=w513:bool)
          }
          frame True {
            n154 = Add(x=w516, y=w520) -> (x+y=w518:dbl)
            n155 = Greater Or Equal?(x=w518, y=w517) -> (x >= y?=w519:bool)
          }
        }
        n156 = call "disable.vi"("error in (no error)"=w508, "Array"=w500) -> ("error out"=w435:errorcluster)  [unwired: 9 in]
        n157 = call "enable.vi"("error in (no error)"=w435, "Array"=w434) -> ("error out"=w433:errorcluster)  [unwired: 9 in]
        n158 = call "field_to_voltage_convert.vi"("Start H Field (Oe)"=w447) -> ("Numeric"=w443:dbl)
        n159 = call-poly <vilib>:"DAQmx Write.vi"("task/channels in"=w473, "data"=w443, "error in"=w433) -> ("task out"=w493:refnum<k21>, "error out"=w492:errorcluster)  [unwired: 10 in, 1 out]
        n160 = flat-sequence {
          tunnel: w439 -> [w556]
          tunnel: w493 -> [w555]
          tunnel: [w555] -> w487
          tunnel: w492 -> [w554]
          tunnel: [w554] -> w491
          tunnel: w472 -> [w553]
          tunnel: [w553] -> w486
          frame #0 {
            n161 = Wait (ms)(milliseconds to wait=w556) -> ()  [unwired: 1 out]
          }
        }
        n162 = call "VNA_measure.vi"("error in (no error)"=w491, "timeout"=w499, "Resource Name In"=w486) -> ("error out"=w498:errorcluster, "Resource Name Out"=w497:refnum<k15>)  [unwired: 7 in]
        n163 = call-poly <instrlib>:"niVNA Fetch.vi"("instrument handle"=w497, "measurement"=w471, "format"=w470, "error in"=w498, "timeout"=w499) -> ("instrument handle out"=w485:refnum<k15>, "data"=w496:dbl[], "error out"=w484:errorcluster)  [unwired: 7 in, 1 out]
        n164 = Add Array Elements(numeric array=w496) -> (sum=w495:dbl)
        n165 = Array Size(array=w496) -> (size(s)=w494:i32)
        n166 = Divide(x=w495, y=w494) -> (x/y=w489:dbl)
        n167 = Unbundle By Name(w468) -> ("Signal"=w490:dbl[], "Field"=w488:dbl[])
        n168 = Build Array (concatenate)(w490, w489) -> (w478:dbl[])
        n169 = Build Array (concatenate)(w488, w447) -> (w477:dbl[])
        n170 = Bundle By Name(cluster=w468, "Signal"=w478, "Field"=w477) -> (w475:T1)
        n171 = Unbundle By Name(w475) -> ("Field"=w463:dbl[], "Signal"=w464:dbl[], "Old Field"=w465:dbl[], "Old Signal"=w466:dbl[])
        n172 = case shown="False" w448 {
          tunnel: [State."Running down" State."Sweeping down"] -> w479
          tunnel: w487 -> [w545 w550]
          tunnel: [w545 w550] -> w483
          tunnel: w485 -> [w544 w551]
          tunnel: [w544 w551] -> w482
          tunnel: w484 -> [w543 w549]
          tunnel: [w543 w549] -> w481
          tunnel: w450 -> [w542 w547]
          tunnel: [w540 w547] -> w480
          tunnel: w475 -> [w539 w548]
          tunnel: [w539 w548] -> w476
          frame False {
            n173 = Add(x=w542, y=1) -> (x+y=w540:i32)
          }
          frame True {
          }
        }
        n174 = Bundle("Field"=w463, "Signal"=w464) -> (w474:cluster{"Field":dbl[], "Signal":dbl[]})  [unwired: 1 in]
        n175 = Bundle("Old Field"=w465, "Old Signal"=w466) -> (w467:cluster{"Old Field":dbl[], "Old Signal":dbl[]})  [unwired: 1 in]
        n176 = Build Array(w474, w467) -> (w444:cluster{"Old Field":dbl[], "Old Signal":dbl[]}[])
        n177 = case shown="True" w469 {
          tunnel: [w528 w537] -> w456
          tunnel: w483 -> [w527 w536]
          tunnel: [w527 w536] -> w457
          tunnel: w482 -> [w526 w535]
          tunnel: [w526 w535] -> w459
          tunnel: w481 -> [w525 w534]
          tunnel: [w525 w534] -> w458
          tunnel: w462 -> [w524 w533]
          tunnel: w480 -> [w523 w532]
          tunnel: [w523 w532] -> w460
          tunnel: w479 -> [w521 _]
          tunnel: [w522 w531] -> w461
          tunnel: w476 -> [w522 w531]
          frame False {
            n178 = Or(x=w525, y=w524) -> (x .or. y?=w529:bool)
            n179 = call "error_check_shutdown_sweep_field.vi"("State In"=w521, "Boolean"=w529) -> ("State Out"=w528:T2)  [unwired: 9 in]
          }
          frame True {
            n180 = Or(x=w534, y=w533) -> (x .or. y?=w538:bool)
            n181 = call "error_check_shutdown_sweep_field.vi"("State In"=State."Sweeping down", "Boolean"=w538) -> ("State Out"=w537:T2)  [unwired: 9 in]
          }
        }
      }
      frame "Shutdown" {
        w577 = T3 3 items=["no dialog", "OK message", "continue or stop message", "OK message + warnings", "continue/stop + warnings"] ("type of dialog (OK msg:1)")
        n182 = control-ref of="Status"() -> (w584:refnum<vi>)
        n183 = call "change_status.vi"("error in (no error)"=w583, "String"="Shutting down...Sweeping field to zero...", "String in"=w584) -> ("error out"=w590:errorcluster)  [unwired: 8 in]
        n184 = call "disable.vi"("error in (no error)"=w590, "Array"=w588) -> ("error out"=w593:errorcluster)  [unwired: 9 in]
        n185 = call "disable.vi"("error in (no error)"=w593, "Array"=w587) -> ("error out"=w592:errorcluster)  [unwired: 9 in]
        n186 = call "disable.vi"("error in (no error)"=w592, "Array"=w586) -> ("error out"=w591:errorcluster)  [unwired: 9 in]
        n187 = call "disable.vi"("error in (no error)"=w591, "Array"=w585) -> ("error out"=w559:errorcluster)  [unwired: 9 in]
        n188 = call "disable.vi"("error in (no error)"=w559, "Array"=w558) -> ("error out"=w557:errorcluster)  [unwired: 9 in]
        n189 = call-poly <vilib>:"DAQmx Write.vi"("task/channels in"=w573, "data"=0.0, "error in"=w557) -> ("task out"=w571:refnum<k21>, "error out"=w572:errorcluster)  [unwired: 10 in, 1 out]
        n190 = Wait (ms)(milliseconds to wait=u32 1000) -> ()  [unwired: 1 out]
        n191 = call <vilib>:"DAQmx Stop Task.vi"("task/channels in"=w571, "error in"=w572) -> ("task out"=w579:refnum<k21>, "error out"=w581:errorcluster)  [unwired: 12 in]
        n192 = call <vilib>:"DAQmx Clear Task.vi"("task in"=w579, "error in"=w581) -> ("error out"=w569:errorcluster)  [unwired: 13 in]
        n193 = call <instrlib>:"niVNA Abort.vi"("instrument handle"=w570, "error in"=w569) -> ("instrument handle out"=w580:refnum<k15>, "error out"=w582:errorcluster)  [unwired: 12 in]
        n194 = call <instrlib>:"niVNA Close.vi"("instrument handle"=w580, "error in"=w582) -> ("error out"=w566:errorcluster)  [unwired: 13 in]
        n195 = property on="SpectrumGraph" class="XYGraph (strict)"(error in=w566, "Value"=cluster{"Old Field":dbl[], "Old Signal":dbl[]}[] [] ("SpectrumGraph")) -> (error out=w564:errorcluster)  [unwired: 1 in, 1 out]
        n196 = control-ref of="Status"() -> (w561:refnum<vi>)
        n197 = call "change_status.vi"("error in (no error)"=w564, "String"="Off", "String in"=w561) -> ("error out"=w563:errorcluster)  [unwired: 8 in]
        n198 = call <vilib>:"Simple Error Handler.vi"("type of dialog (OK msg:1)"=w577, "error in (no error)"=w563) -> ("error out"=w578:errorcluster)  [unwired: 3 in, 4 out]
      }
    }
    "SpectrumGraph" <- w38
    n199 = event shown="[2] \"Save Button\": Value Change" {
      selector: _ -> [_ _ _]
      dyn-events: _ -> [_ _ _]
      timeout: 1 -> [_ _ _]
      event Timeout {
        n200 = event-data() -> ()  [unwired: 1 in, 3 out]
      }
      event "SpectrumGraph": Mouse Down {
        n201 = event-data() -> ("CtlRef"=w78:refnum<vi>, "Coords"=w77:T4)  [unwired: 1 in]
        n202 = invoke on="Invoke Node" class="XYGraph (strict)" method="Map Coords To XY"(reference=w78, "Coords"=w77) -> ("Map Coords To XY"=w79:bool, "XY"=w80:cluster{"X":dbl, "Y":dbl})  [unwired: 5 in, 5 out]
        n203 = case shown="True" w79 {
          tunnel: w80 -> [_ w81]
          frame False {
          }
          frame True {
            n204 = property on="Cursor" class="Clust (strict)"("Value"=w81) -> ()  [unwired: 2 in, 2 out]
          }
        }
      }
      event "Save Button": Value Change {
        # "Field\nSignal"
        n205 = event-data() -> ()  [unwired: 1 in, 1 out]
        n206 = control-ref of="SpectrumGraph"() -> (w90:refnum<vi>)
        n207 = property class="XYGraph (strict)"(reference=w90) -> ("Value"=w88:cluster{"Old Field":dbl[], "Old Signal":dbl[]}[])  [unwired: 1 in, 2 out]
        n208 = Index Array(array=w88, index=1) -> (element=w87:cluster{"Old Field":dbl[], "Old Signal":dbl[]})
        n209 = Unbundle(w87) -> ("Old Field"=w83:dbl[], "Old Signal"=w82:dbl[])
        n210 = call "Convert to Dynamic Data"("Array"=w83) -> ("Dynamic Data Type"=w86:dynamicdata)  [unwired: 3 in]
        n211 = call "Convert to Dynamic Data2"("Array"=w82) -> ("Dynamic Data Type"=w85:dynamicdata)  [unwired: 3 in]
        n212 = Merge Signals(w86, w85) -> (w84:dynamicdata)
        n213 = call "Write To Measurement File"("Signals"=w84) -> ()  [unwired: 16 in, 3 out]
      }
    }
    n214 = case shown="True" "Clear button" {
      tunnel: w36 -> [w72 w76]
      tunnel: [w72 w75] -> w35
      frame False {
      }
      frame True {
        n215 = Bundle By Name(cluster=w76, "Old Field"=dbl[] [], "Old Signal"=dbl[] []) -> (w75:T1)
      }
    }
  }
  "Error Out" <- w6
  "VNA Name Out" <- w12
  "DAQ channel Out" <- w11
  "Cursor" <- cluster{"x":dbl, "y":dbl} {"x"=0.0, "y"=0.0} ("Cursor")
